vi "Main Output Messages.vi"(8 "error in":errorcluster, 11 "internal data":T1={"J1939 XNET Settings"={"XNET Database"="", "XNET Cluster"="", "CAN port"="", "Baud rate [Bd]"=0, "J1939 Network Address"=0, "Name"=0, "Termination"=0}, "j1939 queues"={"Processed Outgoing"=refnum, "Process Outgoing"=refnum, "stop notifier"=refnum, "error queue"=refnum, "active dtc"=refnum, "processed inc"=refnum}, "fgv references"={"BAM Buffer"=refnum, "CM Buffer"=refnum, "CM Gen"=refnum, "BAM Gen"=refnum, "Address Claims"=refnum, "RQST"=refnum, "scaling lut"=refnum, "data lut"=refnum, "cyclic scheduler"=refnum}, "frame in"="", "frame out"="", "timing"={"tb to j1939 queue timeout"=100, "j1939 to tb queue timeout"=100, "dtc loop period (ms)"=100, "CAN in loop period (ms)"=100, "process incoming queue timeout (ms)"=100, "Outgoing Write Decimation"=0, "process outgoing loop rate (ms)"=0, "periodic outgoing queue timeout (ms)"=10, "CAN out queue timeout (ms)"=100}}) -> ()   [LabVIEW 2013, in "J1939.lvlib"]
uses:
  J1939.lvlib
  API Types/Internal Data.ctl
  API Types/XNET Settings.ctl
  API Types/Setup Information Cluster.ctl
  API Types/CAN Outgoing Message Cluster.ctl
  API Types/Convert DTCs Cluster.ctl
  <vilib>/xnet/xnet.llb/XNET Frame CAN.ctl
  <vilib>/xnet/xnet.llb/XNET Frame Type CAN.ctl
  TP/TP List References.ctl
  BAM/BAM Buffer Connections List_Ref.ctl
  Connection Mode/Connection Mode Generation Connection Ref.ctl
  BAM/BAM Generation Connections List_Ref.ctl
  LUTs/J1939 Address Table Reference.ctl
  RQST/RQST Lookup Table Reference.ctl
  LUTs/J1939 Conversion Lookup Table Reference.ctl
  LUTs/J1939 Data Lookup Table Reference.ctl
  LUTs/Cyclic Frame Scheduler Lut Reference.ctl
  Configuration/TypeDefs/timing configuration.ctl
  <vilib>/xnet/xnet.llb/XNET Write (Frame CAN).vi
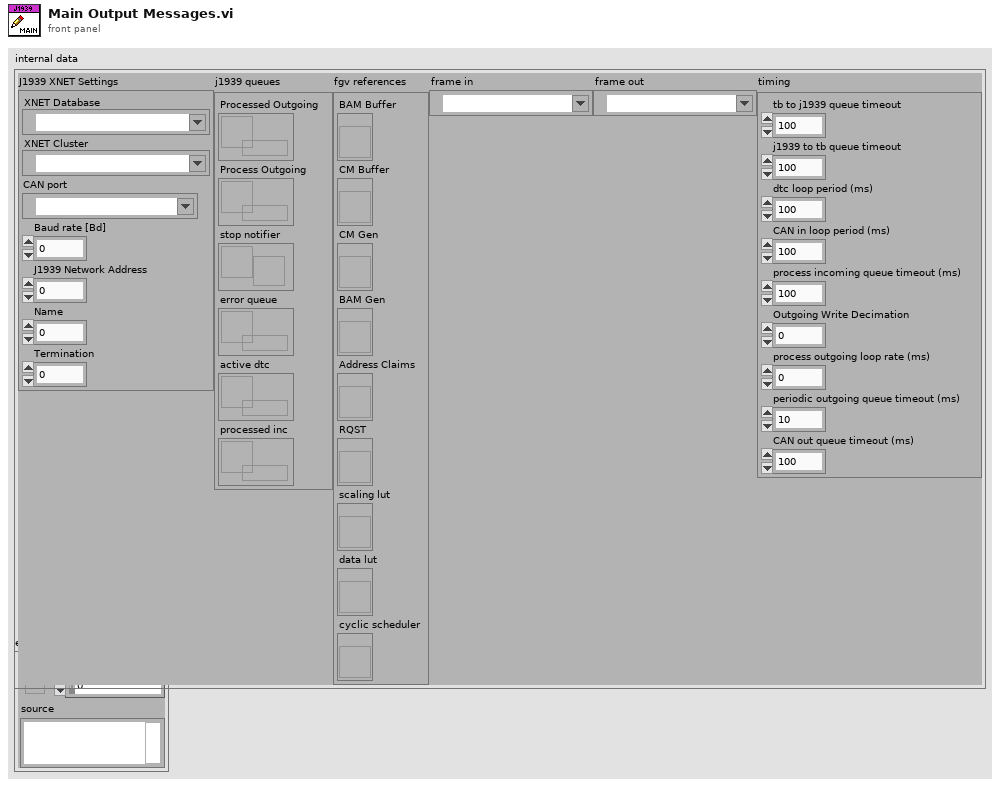
[diagram p1: front panel]
types:
  T1 = typedef "J1939.lvlib/Internal Data.ctl" = cluster{"J1939 XNET Settings":T2, "j1939 queues":T3, "fgv references":T4, "frame in":refnum<k21>, "frame out":refnum<k21>, "timing":T13}
  T2 = typedef "J1939.lvlib/XNET settings.ctl" = cluster{"XNET Database":refnum<k21>, "XNET Cluster":refnum<k21>, "CAN port":refnum<k21>, "Baud rate [Bd]":u32, "J1939 Network Address":u8, "Name":u64, "Termination":u32}
  T3 = typedef "J1939.lvlib/Setup Information Cluster.ctl" = cluster{"Processed Outgoing":refnum<queue>, "Process Outgoing":refnum<queue>, "stop notifier":refnum<notifier>, "error queue":refnum<queue>, "active dtc":refnum<queue>, "processed inc":refnum<queue>}
  T4 = typedef "J1939.lvlib/TP List References.ctl" = cluster{"BAM Buffer":T5, "CM Buffer":T5, "CM Gen":T6, "BAM Gen":T7, "Address Claims":T8, "RQST":T9, "scaling lut":T10, "data lut":T11, "cyclic scheduler":T12}
  T5 = typedef "J1939.lvlib/BAM Buffer Connections List_Ref.ctl" = refnum<vi>
  T6 = typedef "J1939.lvlib/Connection Mode Generation Connection Ref.ctl" = refnum<vi>
  T7 = typedef "J1939.lvlib/BAM Generation Connections List_Ref.ctl" = refnum<vi>
  T8 = typedef "J1939.lvlib/J1939 Address Table Reference.ctl" = refnum<vi>
  T9 = typedef "J1939.lvlib/RQST Lookup Table Reference.ctl" = refnum<vi>
  T10 = typedef "J1939.lvlib/J1939 Conversion Lookup Table Reference.ctl" = refnum<vi>
  T11 = typedef "J1939.lvlib/J1939 Data Lookup Table Reference.ctl" = refnum<vi>
  T12 = typedef "J1939.lvlib/cyclic frame scheduler lut reference.ctl" = refnum<vi>
  T13 = typedef "J1939.lvlib/timing configuration.ctl" = cluster{"tb to j1939 queue timeout":i32, "j1939 to tb queue timeout":i32, "dtc loop period (ms)":i32, "CAN in loop period (ms)":i32, "process incoming queue timeout (ms)":i32, "Outgoing Write Decimation":u32, "process outgoing loop rate (ms)":i32, "periodic outgoing queue timeout (ms)":i32, "CAN out queue timeout (ms)":i32}
  T14 = typedef "J1939.lvlib/CAN Outgoing Message Cluster.ctl" = cluster{"Identifier":u32, "Data":u8[]}
  T15 = typedef "XNET Frame CAN.ctl" = cluster{"timestamp":timestamp, "payload":u8[], "identifier":u32, "type":T16, "extended?":bool, "echo?":bool}
  T16 = typedef "XNET Frame Type CAN.ctl" = u8
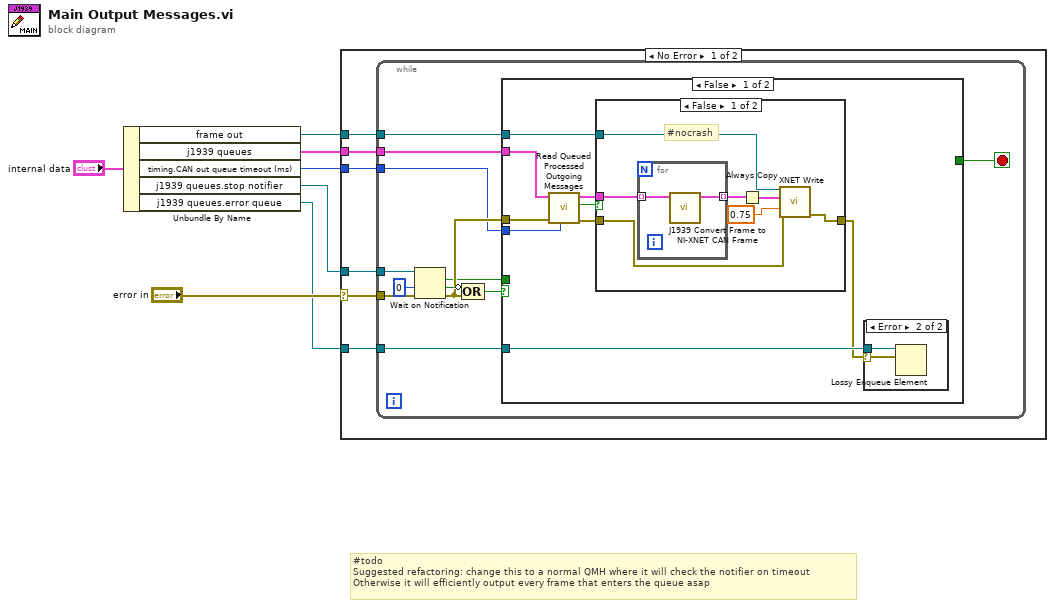
[diagram p0: block diagram]
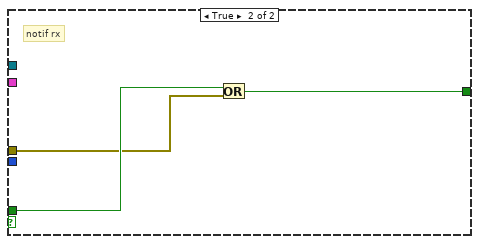
[diagram p4: hidden frame]
diagram:
  # "#todo\nSuggested refactoring: change this to a normal QMH where it will check the notifier on timeout\nOtherwise it will efficiently output every frame that enters the queue asap"
  n1 = Unbundle By Name("internal data") -> ("frame out"=w5:refnum<k21>, "j1939 queues"=w4:T3, "timing.CAN out queue timeout (ms)"=w1:i32, "j1939 queues.stop notifier"=w3:refnum<notifier>, "j1939 queues.error queue"=w2:refnum<queue>)
  n2 = case shown="No Error" "error in" {
    selector: "error in" -> [w13 _]
    tunnel: w3 -> [w12 _]
    tunnel: w5 -> [w11 _]
    tunnel: w4 -> [w10 _]
    tunnel: w2 -> [w9 _]
    tunnel: w1 -> [w8 _]
    frame No Error {
      n3 = while {
        tunnel: w12 -> [w24]
        tunnel: w13 -> [w25]
        tunnel: w11 -> [w17]
        tunnel: w10 -> [w16]
        tunnel: w9 -> [w15]
        tunnel: w8 -> [w14]
        stop <- w19 stop-if-true
        n4 = Wait on Notification(notifier=w24, timeout in ms (-1)=0, error in (no error)=w25) -> (notification=w20:bool, timed out?=w23:bool, error out=w21:errorcluster)  [unwired: 1 in, 1 out]
        n5 = Compound Arithmetic op=OR(invert w23, w21) -> (w22:bool)
        n6 = case shown="False" w22 {
          tunnel: w21 -> [w31 w47]
          tunnel: w20 -> [_ w49]
          tunnel: [_ w48] -> w19
          tunnel: w17 -> [w29 _]
          tunnel: w16 -> [w30 _]
          tunnel: w15 -> [w28 _]
          tunnel: w14 -> [w26 _]
          frame False {
            n7 = call "Read Queued Processed Outgoing Messages.vi"("timeout in ms (-1)"=w26, "error in"=w31, "j1939 queues"=w30) -> ("error out"=w32:errorcluster, "timed out?"=w34:bool, "Frames"=w33:T14[])  [unwired: 6 in]
            n8 = case shown="False" w34 {
              tunnel: w32 -> [w38 w46]
              tunnel: w33 -> [w43 _]
              tunnel: w29 -> [w42 _]
              tunnel: [w41 w46] -> w27
              frame False {
                # "#nocrash"
                n9 = for {
                  tunnel: w43 -> [w45] mode=indexing
                  tunnel: [w44] -> w40 mode=indexing
                  n10 = call "J1939 Convert Frame to NI-XNET CAN Frame.vi"("Data to Send"=w45) -> ("CAN frame"=w44:T15)  [unwired: 1 in, 9 out]
                }
                n11 = Always Copy(1:w40) -> (0:w37:T15[])
                n12 = call-poly <vilib>:"XNET Write.vi"("session in"=w42, "data"=w37, "timeout (10)"=0.75, "error in (no error)"=w38) -> ("error out"=w41:errorcluster)  [unwired: 11 out]
              }
              frame True {
              }
            }
            n13 = case shown="Error" w27 {
              selector: w27 -> [_ w35]
              tunnel: w28 -> [_ w36]
              frame No Error {
              }
              frame Error {
                n14 = Lossy Enqueue Element(queue=w36, element=w35) -> ()  [unwired: 1 in, 4 out]
              }
            }
          }
          frame True {
            # "notif rx"
            n15 = Or(x=w49, y=w47) -> (x .or. y?=w48:bool)
          }
        }
      }
    }
    frame Error {
    }
  }
